vi "Write and Read to the MONO.vi"(4 "MONOCHOMATOR":refnum<visa-resource-name>, 6 "Command":string, 8 "error in":errorcluster) -> (0 "error out":errorcluster, 5 "OUTPUT":string, 7 "VISA resource name out":refnum<visa-resource-name>)   [LabVIEW 2024]
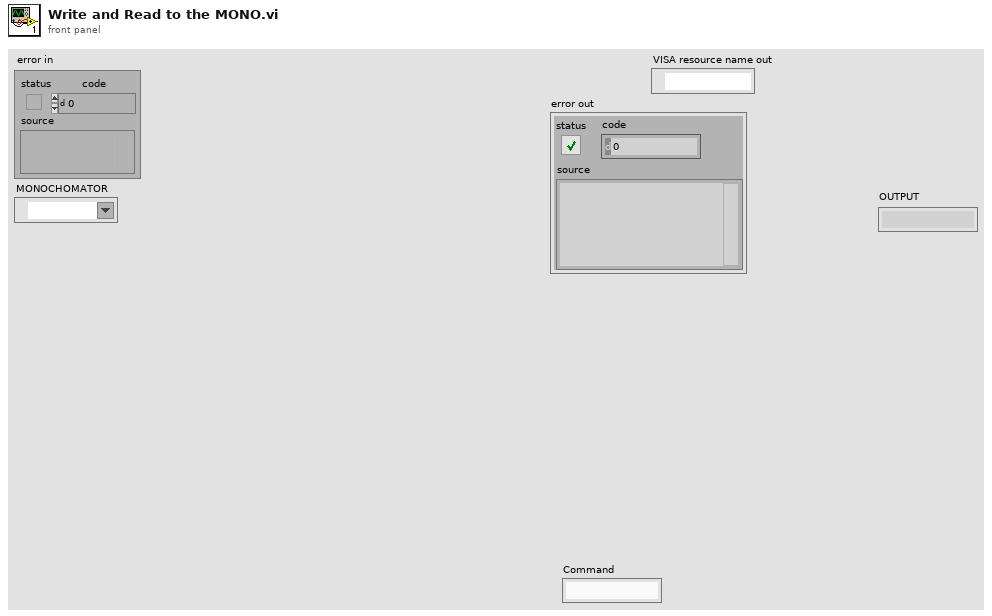
[diagram p1: front panel]
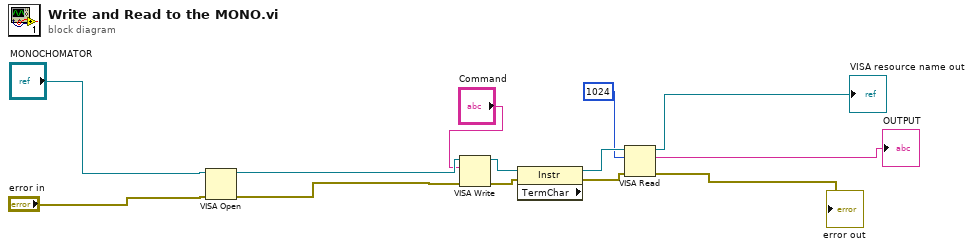
[diagram p0: block diagram]
diagram:
  n1 = VISA Open(error in (no error)="error in", VISA resource name="MONOCHOMATOR") -> (VISA resource name=w13:refnum<visa-resource-name>, error out=w11:errorcluster)  [unwired: 3 in]
  n2 = VISA Write(VISA resource name=w13, write buffer="Command", error in (no error)=w11) -> (VISA resource name out=w7:refnum<visa-resource-name>, error out=w4:errorcluster)  [unwired: 1 out]
  n3 = property class="Instr" props=["TermChar"](reference=w7, error in=w4) -> (reference out=w6:refnum<visa-resource-name>, error out=w5:errorcluster)  [unwired: 1 out]
  n4 = VISA Read(VISA resource name=w6, byte count=u32 1024, error in (no error)=w5) -> (VISA resource name out=→"VISA resource name out":refnum<visa-resource-name>, read buffer=→"OUTPUT":string, error out=→"error out":errorcluster)  [unwired: 1 out]
